vi "StateTransitionEdge_SetModifiedClassAttributes.vi"(0 "reference in":refnum<class "StateTransitionEdge.lvclass">, 2 "Class attributes":T1, 3 "Only unlock data? (F)":bool, 4 "Unlock data if error? (T)":bool=TRUE, 5 "error in (no error)":errorcluster) -> (14 "reference out":refnum<class "StateTransitionEdge.lvclass">, 19 "error out":errorcluster)   [LabVIEW 2012, in "StateTransitionEdge.lvclass"]
doc: "This VI overwrites the class attributes associated with the StateTransitionEdge or subclass object reference and unlocks it for write access. If error in is set, the object is unlocked but its data will not be modified. If reference is wired, the class attributes of the class (or sub class) will be affected else the class attributes will default to the StateTransitionEdge class.\n\nIn order to use this VI, you must first successfully lock the object's data using the StateTransitionEdge GetClassAttributesToModify VI.\n\n[GOOP 2.0.15]"
uses:
  <resource>/Framework/Providers/Open_GDS/UML/StateTransitionEdge_class/StateTransitionEdge.lvclass
  <resource>/Framework/Providers/Open_GDS/UML/StateTransitionEdge_class/protected/ClassAttributes.ctl
  <resource>/Framework/Providers/Open_GDS/UML/ClassRelationshipEdge_class/protected/ClassAttributes.ctl
  <resource>/Framework/Providers/Open_GDS/UML/SegmentedLineEdge_class/protected/ClassAttributes.ctl
  <resource>/Framework/Providers/Open_GDS/UML/GeneralPathEdge_class/protected/ClassAttributes.ctl
  <resource>/Framework/Providers/Open_GDS/UML/AbstractEdge_class/protected/ClassAttributes.ctl
  <vilib>/addons/_goop3.llb/3GOOPStates.ctl
  <resource>/Framework/Providers/Open_GDS/UML/StateTransitionEdge_class/StateTransitionEdge.lvclass/StateTransitionEdge.ctl
  <resource>/Framework/Providers/Open_GDS/UML/AbstractEdge_class/AbstractEdge.lvclass
  <resource>/Framework/Providers/Open_GDS/UML/GeneralPathEdge_class/GeneralPathEdge.lvclass
  <resource>/Framework/Providers/Open_GDS/UML/SegmentedLineEdge_class/SegmentedLineEdge.lvclass
  <resource>/Framework/Providers/Open_GDS/UML/ClassRelationshipEdge_class/ClassRelationshipEdge.lvclass
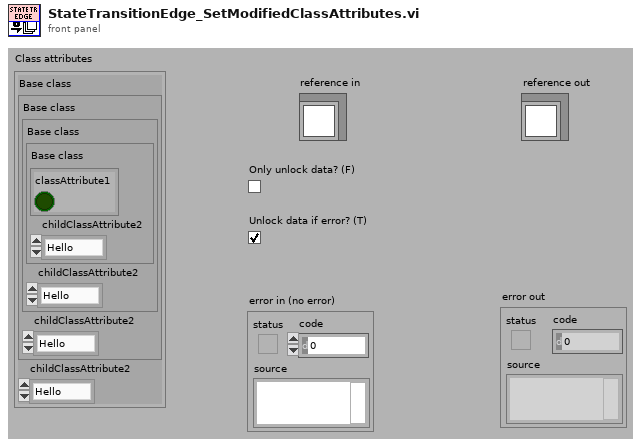
[diagram p1: front panel]
types:
  T1 = typedef "StateTransitionEdge.lvclass/ClassAttributes.ctl" = cluster{"Base class":T2, "childClassAttribute2":enum16{"Hello", "Goodbye"}}
  T2 = typedef "ClassRelationshipEdge.lvclass/ClassAttributes.ctl" = cluster{"Base class":T3, "childClassAttribute2":enum16{"Hello", "Goodbye"}}
  T3 = typedef "SegmentedLineEdge.lvclass/ClassAttributes.ctl" = cluster{"Base class":T4, "childClassAttribute2":enum16{"Hello", "Goodbye"}}
  T4 = typedef "GeneralPathEdge.lvclass/ClassAttributes.ctl" = cluster{"Base class":T5, "childClassAttribute2":enum16{"Hello", "Goodbye"}}
  T5 = typedef "AbstractEdge.lvclass/ClassAttributes.ctl" = cluster{"classAttribute1":bool}
  T6 = typedef "3GOOPStates.ctl" = enum16{"Set", "Get", "New", "Delete", "Clear", "Test and get", "Unlock data", "Information", "Look up existing", "New or look up existing", "Test and get shared", "Get shared", "Set shared", "Unlock shared", "Find dynamic method", "Register dynamic method", "Preload dynamic method", "Probe", "Cast to more generic", "Cast to more specific"}
  T7 = typedef "AbstractEdge.lvclass/ObjectReference.ctl" = refnum<k1>
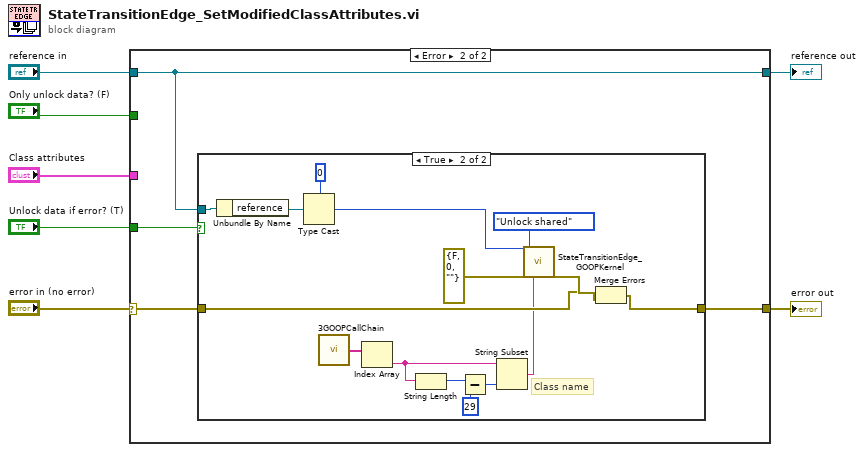
[diagram p0: block diagram]
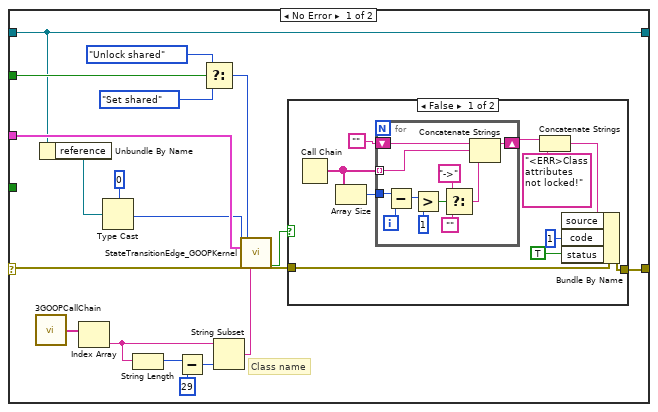
[diagram p2: hidden frame]
diagram:
  n1 = case shown="Error" "error in (no error)" {
    selector: "error in (no error)" -> [w15 w50]
    tunnel: [w21 w49] -> w3
    tunnel: "Class attributes" -> [w25 _]
    tunnel: [w16 w51] -> w6
    tunnel: "reference in" -> [w21 w49]
    tunnel: "Only unlock data? (F)" -> [w26 _]
    tunnel: "Unlock data if error? (T)" -> [_ w52]
    frame No Error {
      # "Class name"
      n2 = call <vilib>:"3GOOPCallChain.vi"() -> ("call chain"=w13:string[])
      n3 = Unbundle By Name(w21) -> ("reference"=w8:T7)
      n4 = Index Array(array=w13) -> (element=w10:string)  [unwired: 1 in]
      n5 = Type Cast(type=0, x=w8) -> (*(type *) &x=w19:i32)
      n6 = String Length(string=w10) -> (length=w14:i32)
      n7 = Subtract(x=w14, y=29) -> (x-y=w12:i32)
      n8 = Select(t=3GOOPStates."Unlock shared" ("Action"), s=w26, f=3GOOPStates."Set shared" ("Action")) -> (s? t:f=w22:T6)
      n9 = String Subset(string=w10, length (rest)=w12) -> (substring=w9:string)  [unwired: 1 out]
      n10 = call <resource>:"StateTransitionEdge_GOOPKernel.vi"("Ref in"=w19, "Data shared in"=w25, "error in (no error)"=w15, "Action"=w22, "Dynamic VI name"=w9) -> ("Data locked?"=w17:bool, "error out"=w18:errorcluster)  [unwired: 10 in, 11 out]
      n11 = case shown="False" w17 {
        tunnel: w18 -> [w31 w48]
        tunnel: [w32 w48] -> w16
        frame False {
          n12 = Call Chain() -> (call chain=w27:string[])
          n13 = Array Size(array=w27) -> (size(s)=w35:i32)
          n14 = for {
            shift-right: [w41] -> w34
            shift-left: "" -> [w43]
            tunnel: w27 -> [w42] mode=indexing
            tunnel: w35 -> [w47]
            i -> [w46]
            n15 = Subtract(x=w47, y=w46) -> (x-y=w45:i32)
            n16 = Greater?(x=w45, y=1) -> (0:w38:bool)
            n17 = Select(t="->", s=w38, f="") -> (s? t:f=w37:string)
            n18 = Concatenate Strings(w43, w42, w37) -> (w41:string)
          }
          n19 = Concatenate Strings(w34, "<ERR>Class attributes not locked!" ("Bundle Element")) -> (w30:string)
          n20 = Bundle By Name(cluster=w31, "source"=w30, "code"=1, "status"=TRUE) -> (w32:errorcluster)
        }
        frame True {
        }
      }
    }
    frame Error {
      n21 = case shown="True" w52 {
        tunnel: w50 -> [w53 w62]
        tunnel: [w53 w64] -> w51
        tunnel: w49 -> [_ w66]
        frame False {
        }
        frame True {
          # "Class name"
          n22 = Unbundle By Name(w66) -> ("reference"=w60:T7)
          n23 = Type Cast(type=0, x=w60) -> (*(type *) &x=w67:i32)
          n24 = call <vilib>:"3GOOPCallChain.vi"() -> ("call chain"=w58:string[])
          n25 = Index Array(array=w58) -> (element=w55:string)  [unwired: 1 in]
          n26 = String Length(string=w55) -> (length=w59:i32)
          n27 = Subtract(x=w59, y=29) -> (x-y=w57:i32)
          n28 = String Subset(string=w55, length (rest)=w57) -> (substring=w54:string)  [unwired: 1 out]
          n29 = call <resource>:"StateTransitionEdge_GOOPKernel.vi"("Ref in"=w67, "error in (no error)"=errorcluster {"status"=FALSE, "code"=0, "source"=""}, "Action"=3GOOPStates."Unlock shared", "Dynamic VI name"=w54) -> ("error out"=w63:errorcluster)  [unwired: 11 in, 12 out]
          n30 = Merge Errors(w62, w63) -> (w64:errorcluster)
        }
      }
    }
  }
  "error out" <- w6
  "reference out" <- w3
